vi "writeDM_Zernike_v2.vi"(1 "amplitude":dbl[](array[numeric])) -> (0 "V Map Out":dbl[][](array[numeric]))   [LabVIEW 2015]
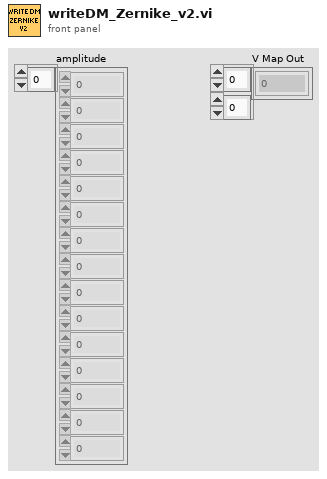
[diagram p1: front panel]
types:
  T1 = typedef "AbberationControl.ctl" = cluster{"Abberations":dbl[][], "Modes":i32[], "Flat":dbl[], "Abberations ID":string[][]}
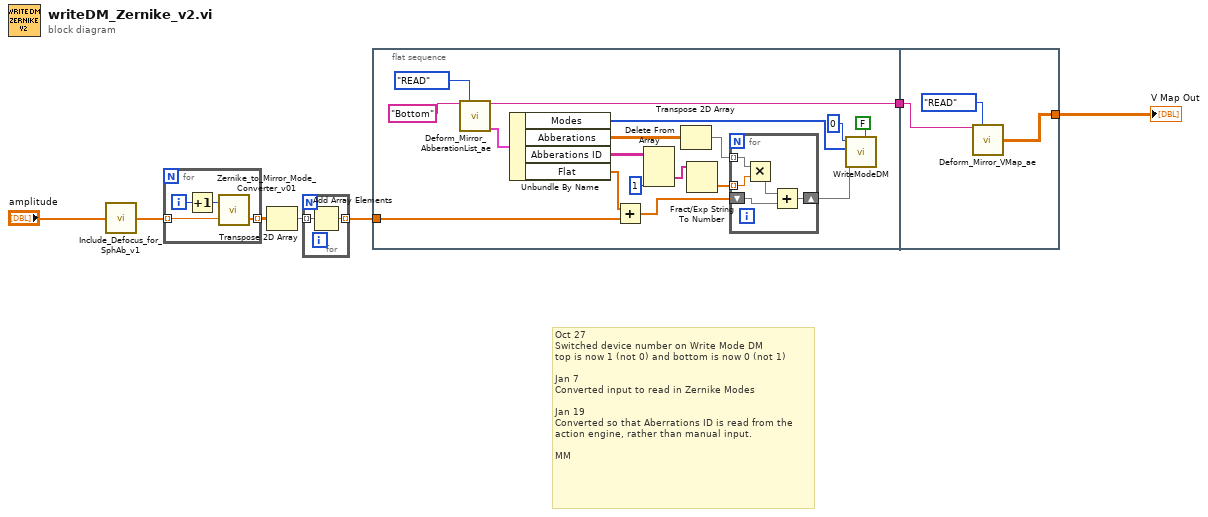
[diagram p0: block diagram]
diagram:
  # "Oct 27\nSwitched device number on Write Mode DM\ntop is now 1 (not 0) and bottom is now 0 (not 1)\n\nJan 7\nConverted input to read in Zernike Modes\n\nJan 19\nConverted so that Aberrations ID is read from the\naction engine, rather than manual input.\n\nMM"
  n1 = call "Include_Defocus_for_SphAb_v1.vi"("amplitude in"="amplitude") -> ("amplitude out"=w1:dbl[])
  n2 = for {
    tunnel: w1 -> [w11] mode=indexing
    tunnel: [w8] -> w6 mode=indexing
    i -> [w10]
    n3 = Increment(x=w10) -> (x+1=w9:i32)
    n4 = call "Zernike_to_Mirror_Mode_Converter_v01.vi"("Zernike Mode Amplitude"=w11, "Zernike Mode"=w9) -> ("Mirror Mode Amplitude"=w8:dbl[])  [unwired: 1 out]
  }
  n5 = Transpose 2D Array(2D array=w6) -> (transposed array=w5:dbl[][])
  n6 = for {
    tunnel: w5 -> [w13] mode=indexing
    tunnel: [w12] -> w4 mode=indexing
    n7 = Add Array Elements(numeric array=w13) -> (sum=w12:dbl)
  }
  n8 = flat-sequence {
    tunnel: w4 -> [w23]
    tunnel: [w20] -> w3
    tunnel: w3 -> [w37]
    tunnel: [w36] -> w7
    frame #0 {
      n9 = call "Deform_Mirror_AbberationList_ae.vi"("Mirror ID"="Bottom", "Enum"=enum16{"WRITE", "READ"}."READ") -> ("Mirror ID Out"=w20:string, "Abberation Cluster Out"=w28:T1)  [unwired: 12 in]
      n10 = Unbundle By Name(w28) -> ("Modes"=w25:i32[], "Abberations"=w16:dbl[][], "Abberations ID"=w17:string[][], "Flat"=w21:dbl[])
      n11 = Add(x=w21, y=w23) -> (x+y=w22:dbl[])
      n12 = Delete From Array(array=w17, index (col)=1 ("index")) -> (deleted portion=w19:string[])  [unwired: 2 in, 1 out]
      n13 = Transpose 2D Array(2D array=w16) -> (transposed array=w15:dbl[][])
      n14 = Fract/Exp String To Number(string=w19) -> (number=w14:dbl[])  [unwired: 3 in, 1 out]
      n15 = for {
        shift-right: [w31] -> w24
        shift-left: w22 -> [w33]
        tunnel: w15 -> [w35] mode=indexing
        tunnel: w14 -> [w34] mode=indexing
        n16 = Multiply(x=w35, y=w34) -> (x*y=w32:dbl[])
        n17 = Add(x=w32, y=w33) -> (x+y=w31:dbl[])
      }
      n18 = call "WriteModeDM.vi"("ClearV"=FALSE, "Amplitudes"=w24, "Modes"=w25, "Device"=0) -> ()  [unwired: 7 in, 1 out]
    }
    frame #1 {
      n19 = call "Deform_Mirror_VMap_ae.vi"("Mirror ID"=w37, "Enum"=enum16{"WRITE", "READ"}."READ") -> ("V Map Out"=w36:dbl[][])  [unwired: 13 in]
    }
  }
  "V Map Out" <- w7
